vi "Write Assert Factory.vi"(8 "error in (no error)":errorcluster, 11 "Assert Factory":refnum<class "Assert Factory.lvclass">) -> (0 "error out":errorcluster)   [LabVIEW 2009, in "Caraya.lvlib" / "Assert Factory Global.lvclass"]
uses:
  Assert Factory Global.lvclass
  Assert Factory/Assert Factory.lvclass
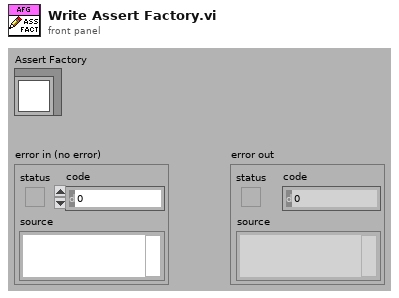
[diagram p1: front panel]
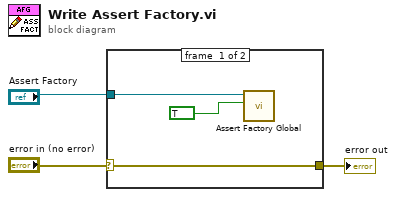
[diagram p0: block diagram]
diagram:
  n1 = case shown="No Error" "error in (no error)" {
    selector: "error in (no error)" -> [w4 w7]
    tunnel: "Assert Factory" -> [w6 _]
    tunnel: [w4 w7] -> w1
    frame #0 {
      n2 = call "Assert Factory Global.vi"("Set (F)"=TRUE, "Assert Factory in"=w6) -> ()  [unwired: 7 in, 3 out]
    }
    frame #1 {
    }
  }
  "error out" <- w1
